vi "CO Serial Data Driver.vi"() -> ()   [LabVIEW 2014]
uses:
  <vilib>/Instr/_visa.llb/VISA Configure Serial Port (Instr).vi
panel:
  in  "Command":string="CONC?"
  in  "VISA resource name 2":refnum<visa-resource-name>="ASRL8::INSTR"
  out ">100msec counter":u32
  out "Receive Time taken history":u32(graph)
  out "Max Receive Time":u32
  out "Command":string
  out "RAW DATA":string
  out "Time taken history":u32(graph)
  out "Max Acq Time diff":u32
  out "Acq Time":u32
  out "loop count":i32
  out "Number of error":i32
  in  "milliseconds to wait":u32=320
  out "Command In":string
  out "error out":errorcluster
  # "COM1 FOR LABVIEW LAPTOP\nCOM2 FOR PCLJ"
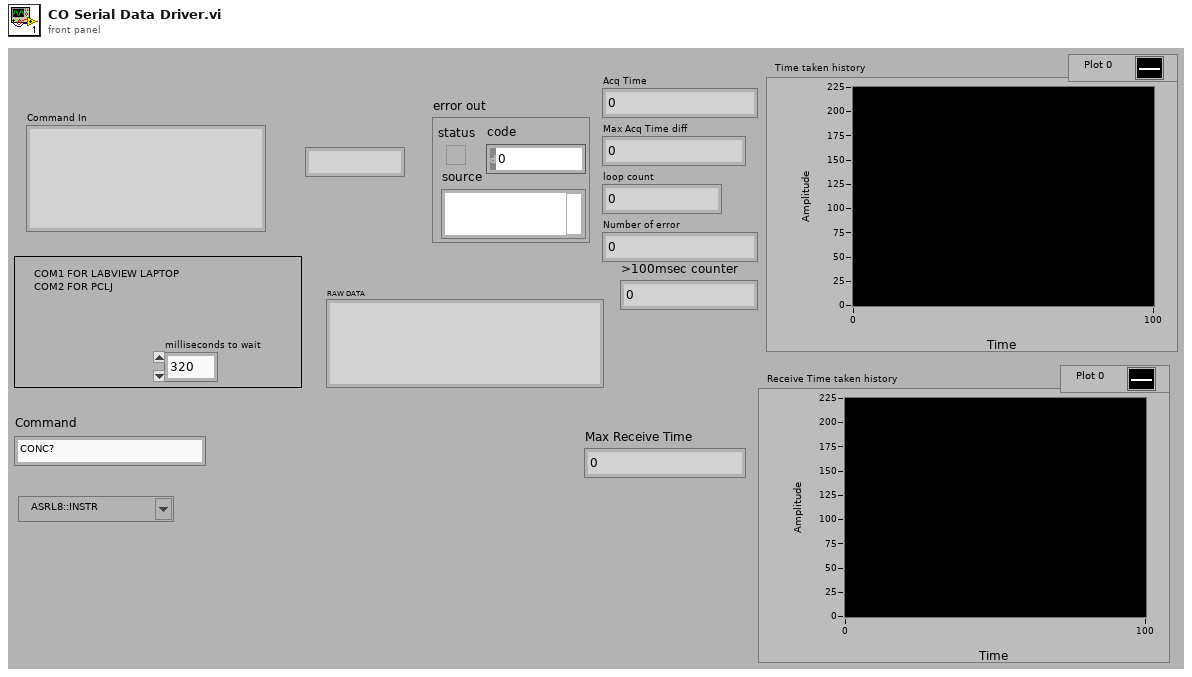
[diagram p1: front panel]
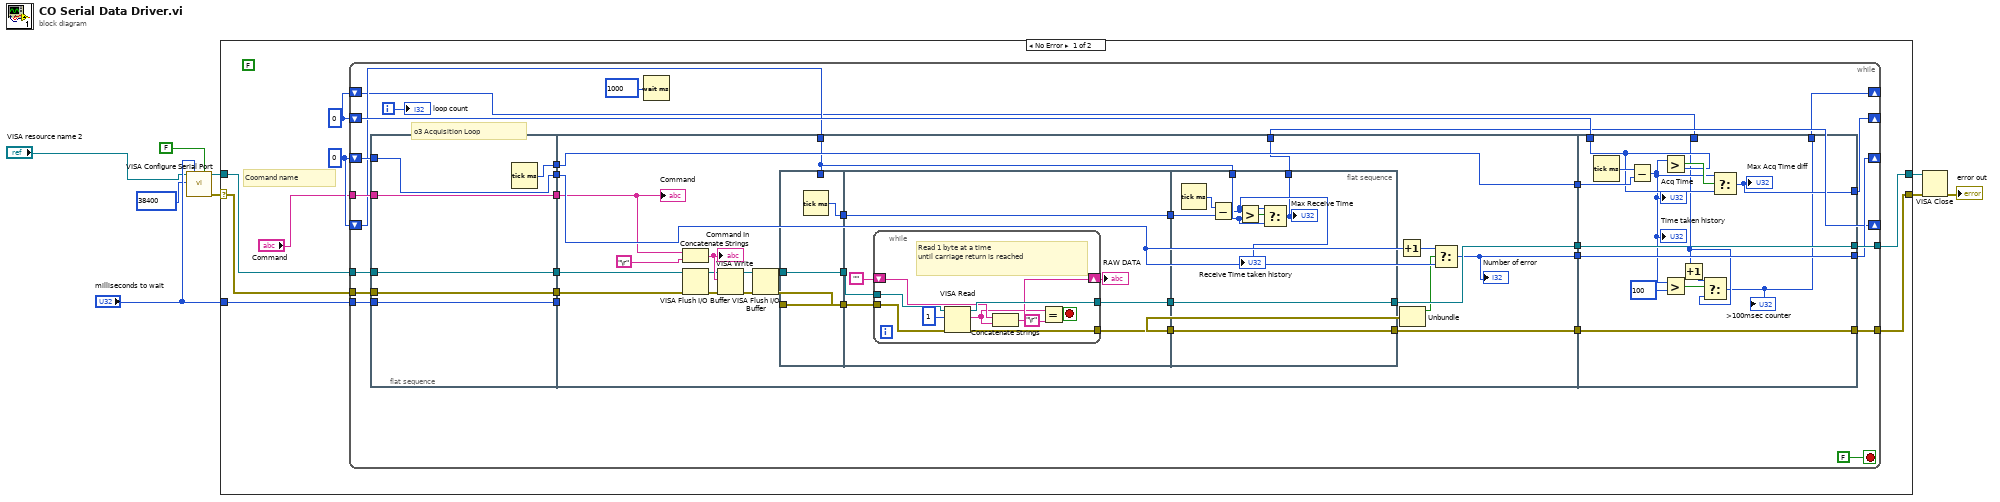
[diagram p0: block diagram]
diagram:
  n1 = call-poly "VISA Configure Serial Port"("VISA resource name"="VISA resource name 2", "timeout (10sec)"="milliseconds to wait", "Enable Termination\nChar (T)"=FALSE ("Enable Termination\nChar (T)"), "baud rate (9600)"=u32 38400) -> ("VISA resource name out"=w9:refnum<visa-resource-name>, "error out"=w4:errorcluster)  [unwired: 10 in]
  n2 = case shown="No Error" w4 {
    selector: w4 -> [w13 w119]
    tunnel: w9 -> [w14 w120]
    tunnel: [w16 w120] -> w7
    tunnel: [w17 w119] -> w6
    tunnel: "milliseconds to wait" -> [w15 _]
    frame No Error {
      (unwired) FALSE ("stop")
      w11 = u32 0
      w12 = u32 0
      # "Coomand name"
      n3 = while {
        tunnel: w14 -> [w44]
        tunnel: w13 -> [w43]
        tunnel: [w42] -> w17
        tunnel: [w41] -> w16
        shift-right: [w37] -> _
        shift-left: w12 -> [w39]
        tunnel: "Command" -> [w38]
        tunnel: w15 -> [w36]
        shift-right: [w24] -> _
        shift-left: w11 -> [w25]
        shift-right: [w21] -> _
        shift-left: w12 -> [w22]
        shift-right: [w19] -> _
        shift-left: w11 -> [w20]
        i -> [w40]
        stop <- FALSE stop-if-true
        # "o3 Acquisition Loop"
        n4 = flat-sequence {
          tunnel: w36 -> [w46]
          tunnel: w38 -> [w47]
          tunnel: w39 -> [w48]
          tunnel: w43 -> [w49]
          tunnel: w44 -> [w50]
          tunnel: [w50] -> w32
          tunnel: [w49] -> w31
          tunnel: [w48] -> w30
          tunnel: [w47] -> w29
          tunnel: [w46] -> w28
          tunnel: [w45] -> w26
          tunnel: [w74] -> w35
          tunnel: [w73] -> w34
          tunnel: [w71] -> w33
          tunnel: w32 -> [w76]
          tunnel: w31 -> [w75]
          tunnel: w30 -> [w72]
          tunnel: w29 -> [w59]
          tunnel: w28 -> [_]
          tunnel: [w70] -> w27
          tunnel: w26 -> [w70]
          tunnel: w22 -> [w52]
          tunnel: [w51] -> w21
          tunnel: [w116] -> w37
          tunnel: [w117] -> w41
          tunnel: [w118] -> w42
          tunnel: w35 -> [w118]
          tunnel: w34 -> [w117]
          tunnel: w33 -> [w116]
          tunnel: w27 -> [w113]
          tunnel: w25 -> [w112]
          tunnel: [w111] -> w24
          tunnel: w20 -> [w106]
          tunnel: [w105] -> w19
          frame #0 {
            n5 = Tick Count (ms)() -> (millisecond timer value=w45:u32)
          }
          frame #1 {
            n6 = Concatenate Strings(w59, "\r") -> (w66:string)
            "Command In" <- w66
            n7 = VISA Flush I/O Buffer(VISA resource name=w76, error in (no error)=w75) -> (VISA resource name out=w65:refnum<visa-resource-name>, error out=w64:errorcluster)  [unwired: 1 in]
            n8 = VISA Write(VISA resource name=w65, write buffer=w66, error in (no error)=w64) -> (VISA resource name out=w67:refnum<visa-resource-name>, error out=w68:errorcluster)  [unwired: 1 out]
            n9 = VISA Flush I/O Buffer(VISA resource name=w67, error in (no error)=w68) -> (VISA resource name out=w61:refnum<visa-resource-name>, error out=w60:errorcluster)  [unwired: 1 in]
            n10 = flat-sequence {
              tunnel: w60 -> [w78]
              tunnel: w61 -> [w79]
              tunnel: [w79] -> w58
              tunnel: [w78] -> w57
              tunnel: w52 -> [_]
              tunnel: [w77] -> w53
              tunnel: w58 -> [w82]
              tunnel: w57 -> [w81]
              tunnel: [w86] -> w56
              tunnel: [w85] -> w55
              tunnel: [w80] -> w54
              tunnel: w53 -> [w80]
              tunnel: [w103] -> w73
              tunnel: [w104] -> w74
              tunnel: w56 -> [w104]
              tunnel: w55 -> [w103]
              tunnel: w54 -> [w101]
              tunnel: w52 -> [w99]
              tunnel: [w97] -> w51
              frame #0 {
                n11 = Tick Count (ms)() -> (millisecond timer value=w77:u32)
              }
              frame #1 {
                n12 = while {
                  tunnel: [w96] -> w85
                  tunnel: [w95] -> w86
                  tunnel: w82 -> [w94]
                  tunnel: w81 -> [w93]
                  shift-right: [w91] -> w83
                  shift-left: "" -> [w92]
                  stop <- w88 stop-if-true
                  # "Read 1 byte at a time \nuntil carriage return is reached"
                  n13 = VISA Read(VISA resource name=w94, byte count=u32 1, error in (no error)=w93) -> (VISA resource name out=w96:refnum<visa-resource-name>, read buffer=w90:string, error out=w95:errorcluster)  [unwired: 1 out]
                  n14 = Concatenate Strings(w92, w90) -> (w91:string)
                  n15 = Equal?(x=w90, y="\r") -> (x = y?=w88:bool)
                }
                "RAW DATA" <- w83
              }
              frame #2 {
                n16 = Tick Count (ms)() -> (millisecond timer value=w102:u32)
                n17 = Subtract(x=w102, y=w101) -> (x-y=w98:u32)
                "Receive Time taken history" <- w98
                n18 = Greater?(x=w98, y=w99) -> (0:w100:bool)
                n19 = Select(t=w98, s=w100, f=w99) -> (s? t:f=w97:u32)
                "Max Receive Time" <- w97
              }
            }
            n20 = Increment(x=w72) -> (x+1=w62:u32)
            n21 = Unbundle(w74) -> ("status"=w63:bool)  [unwired: 2 out]
            n22 = Select(t=w62, s=w63, f=w72) -> (s? t:f=w71:u32)
            "Number of error" <- w71
            "Command" <- w59
          }
          frame #2 {
            n23 = Tick Count (ms)() -> (millisecond timer value=w115:u32)
            n24 = Subtract(x=w115, y=w113) -> (x-y=w110:u32)
            "Acq Time" <- w110
            "Time taken history" <- w110
            n25 = Greater?(x=w110, y=w112) -> (0:w114:bool)
            n26 = Greater?(x=w110, y=u32 100) -> (0:w108:bool)
            n27 = Increment(x=w106) -> (x+1=w107:u32)
            n28 = Select(t=w107, s=w108, f=w106) -> (s? t:f=w105:u32)
            ">100msec counter" <- w105
            n29 = Select(t=w110, s=w114, f=w112) -> (s? t:f=w111:u32)
            "Max Acq Time diff" <- w111
          }
        }
        n30 = Wait (ms)(milliseconds to wait=u32 1000) -> ()  [unwired: 1 out]
        "loop count" <- w40
      }
    }
    frame Error {
    }
  }
  n31 = VISA Close(VISA resource name=w7, error in (no error)=w6) -> (error out=→"error out":errorcluster)
